vi "Test Read DAT and TDMS.vi"() -> ()   [LabVIEW 2019]
uses:
  3811ab8e-563b-4f0e-ab82-2145b4b5b4ca.vi
  9b17270d-5d0c-4365-9a1f-7ea8eb203ad9.vi
  6996a507-959e-4011-8723-71fb57f9d81e.vi
  06af5cf2-6c13-4970-920c-06c6a4bda324.vi
  0d41830b-9568-4bf9-b5e1-5d65a9571d75.vi
  1d0c72e7-2fd5-4ada-9d2c-d8c7b4a58351.vi
  <userlib>/_OpenG.lib/file/file.llb/Build Path - File Names Array__ogtk.vi
  <vilib>/Utility/error.llb/Error Cluster From Error Code.vi
  LV-Data/LV-Data.lvclass
panel:
  in  "TDMS Folder":path=path "G:/.shortcut-targets-by-id/0B8-gGFa6hkR4XzJJMDlqZXVKRk0/ansom/Data/MNK/SA40379A.20221206/01 - Vtg test"
  in  "TDMS File":path=path "G:/.shortcut-targets-by-id/0B8-gGFa6hkR4XzJJMDlqZXVKRk0/ansom/Data/PPMSDAQ/2020/PPMS 1/SA40244A.20210723/03-Sweep B IV/SA40244A.20210723.000000.tdms"
  in  "DAT file":path=path "G:/.shortcut-targets-by-id/0B8-gGFa6hkR4XzJJMDlqZXVKRk0/ansom/Data/MNK/SA40286K.20220307/00-Cooldown/SA40286K.20220307.000000.dat"
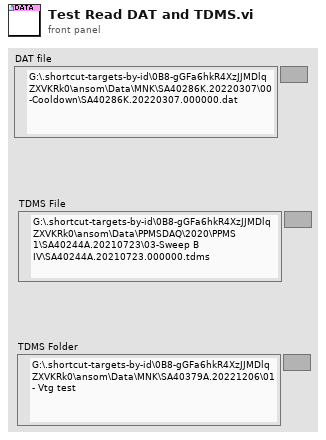
[diagram p1: front panel]
types:
  T1 = typedef "LV-Data.lvclass/Dictionary--cluster.ctl" = cluster{"key":string, "value":variant}
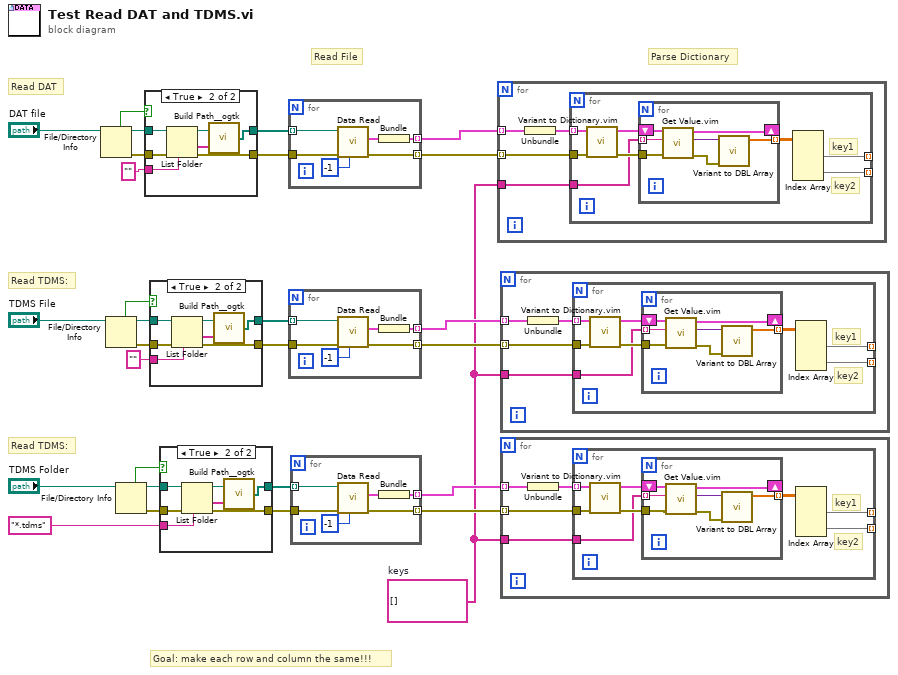
[diagram p0: block diagram]
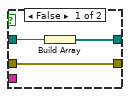
[diagram p2: hidden frame]
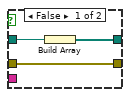
[diagram p3: hidden frame]
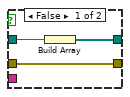
[diagram p4: hidden frame]
diagram:
  w16 = string[] []  # keys
  # "Goal: make each row and column the same!!!"
  # "Parse Dictionary"
  # "Read File"
  # "Read DAT"
  # "Read TDMS:"
  # "Read TDMS:"
  n1 = File/Directory Info(path="DAT file") -> (path out=w10:path, directory=w8:bool, error out=w9:errorcluster)  [unwired: 1 in, 4 out]
  n2 = File/Directory Info(path="TDMS File") -> (path out=w12:path, directory=w14:bool, error out=w13:errorcluster)  [unwired: 1 in, 4 out]
  n3 = File/Directory Info(path="TDMS Folder") -> (path out=w27:path, directory=w15:bool, error out=w25:errorcluster)  [unwired: 1 in, 4 out]
  n4 = case shown="True" w8 {
    tunnel: w10 -> [w31 w38]
    tunnel: [w30 w37] -> w5
    tunnel: w9 -> [w29 w36]
    tunnel: [w29 w35] -> w4
    tunnel: "" ("pattern") -> [_ w34]
    frame False {
      n5 = Build Array(w31) -> (w30:path[])
    }
    frame True {
      n6 = List Folder(path=w38, pattern=w34, error in=w36) -> (path out=w33:path, folder names=w32:string[], error out=w35:errorcluster)  [unwired: 1 in, 1 out]
      n7 = call-poly <userlib>:"Build Path__ogtk.vi"("name or relative path"=w32, "base path"=w33) -> ("appended path"=w37:path[])
    }
  }
  n8 = case shown="True" w14 {
    tunnel: w12 -> [w41 w48]
    tunnel: [w40 w47] -> w11
    tunnel: w13 -> [w39 w46]
    tunnel: [w39 w45] -> w3
    tunnel: "" ("pattern") -> [_ w44]
    frame False {
      n9 = Build Array(w41) -> (w40:path[])
    }
    frame True {
      n10 = List Folder(path=w48, pattern=w44, error in=w46) -> (path out=w43:path, folder names=w42:string[], error out=w45:errorcluster)  [unwired: 1 in, 1 out]
      n11 = call-poly <userlib>:"Build Path__ogtk.vi"("name or relative path"=w42, "base path"=w43) -> ("appended path"=w47:path[])
    }
  }
  n12 = case shown="True" w15 {
    tunnel: w27 -> [w51 w58]
    tunnel: [w50 w57] -> w26
    tunnel: w25 -> [w49 w56]
    tunnel: [w49 w55] -> w24
    tunnel: "*.tdms" ("pattern") -> [_ w54]
    frame False {
      n13 = Build Array(w51) -> (w50:path[])
    }
    frame True {
      n14 = List Folder(path=w58, pattern=w54, error in=w56) -> (path out=w53:path, folder names=w52:string[], error out=w55:errorcluster)  [unwired: 1 in, 1 out]
      n15 = call-poly <userlib>:"Build Path__ogtk.vi"("name or relative path"=w52, "base path"=w53) -> ("appended path"=w57:path[])
    }
  }
  n16 = for {
    tunnel: w5 -> [w64] mode=indexing
    tunnel: [w61] -> w17 mode=indexing
    tunnel: [w60] -> w18 mode=indexing
    tunnel: w4 -> [w59]
    n17 = call "Data Read.vi"("Append Index"=-1, "error in (no error)"=w59, "path"=w64) -> ("error out"=w60:errorcluster, "Data (Dictionary)"=w62:T1[])  [unwired: 5 in, 2 out]
    n18 = Bundle("Data (Dictionary)"=w62) -> (w61:cluster{"Data (Dictionary)":T1[]})  [unwired: 1 in]
  }
  n19 = for {
    tunnel: w11 -> [w70] mode=indexing
    tunnel: [w67] -> w19 mode=indexing
    tunnel: [w66] -> w20 mode=indexing
    tunnel: w3 -> [w65]
    n20 = call "Data Read.vi"("Append Index"=-1, "error in (no error)"=w65, "path"=w70) -> ("error out"=w66:errorcluster, "Data (Dictionary)"=w68:T1[])  [unwired: 5 in, 2 out]
    n21 = Bundle("Data (Dictionary)"=w68) -> (w67:cluster{"Data (Dictionary)":T1[]})  [unwired: 1 in]
  }
  n22 = for {
    tunnel: w26 -> [w76] mode=indexing
    tunnel: w24 -> [w75]
    tunnel: [w73] -> w22 mode=indexing
    tunnel: [w71] -> w21 mode=indexing
    n23 = call "Data Read.vi"("Append Index"=-1, "error in (no error)"=w75, "path"=w76) -> ("error out"=w71:errorcluster, "Data (Dictionary)"=w72:T1[])  [unwired: 5 in, 2 out]
    n24 = Bundle("Data (Dictionary)"=w72) -> (w73:cluster{"Data (Dictionary)":T1[]})  [unwired: 1 in]
  }
  n25 = for {
    tunnel: w17 -> [w80] mode=indexing
    tunnel: w18 -> [w78] mode=indexing
    tunnel: w16 -> [w77]
    n26 = Unbundle(w80) -> ("Data (Dictionary)"=w79:T1[])
    n27 = for {
      tunnel: w79 -> [w87] mode=indexing
      tunnel: [w85] -> _ mode=indexing
      tunnel: [w84] -> _ mode=indexing
      tunnel: w78 -> [w83]
      tunnel: w77 -> [w81]
      # "key2"
      # "key1"
      n28 = call "Variant to Dictionary.vim"("error in (no error)"=w83, "key-value"=w87) -> ("error out"=w82:errorcluster, "Dictionary"=w88:T1[])  [unwired: 8 in]
      n29 = for {
        tunnel: w81 -> [w93] mode=indexing
        shift-right: [w91] -> _
        shift-left: w88 -> [w92]
        tunnel: [w90] -> w86 mode=indexing
        tunnel: w82 -> [w89]
        n30 = call "Get Value.vim"("error in (no error)"=w89, "Key"=w93, "map in"=w92) -> ("error out"=w94:errorcluster, "value"=w95:variant, "map out"=w91:T1[])  [unwired: 6 in]
        n31 = call "Variant to DBL Array.vi"("error in (no error)"=w94, "Data (Variant)"=w95) -> ("1D Array"=w90:dbl[])  [unwired: 7 in, 2 out]
      }
      n32 = Index Array(array=w86) -> (element #1=w85:dbl[], element #2=w84:dbl[])  [unwired: 4 in]
    }
  }
  n33 = for {
    tunnel: w19 -> [w99] mode=indexing
    tunnel: w20 -> [w97] mode=indexing
    tunnel: w16 -> [w96]
    n34 = Unbundle(w99) -> ("Data (Dictionary)"=w98:T1[])
    n35 = for {
      tunnel: w98 -> [w106] mode=indexing
      tunnel: [w104] -> _ mode=indexing
      tunnel: [w103] -> _ mode=indexing
      tunnel: w97 -> [w102]
      tunnel: w96 -> [w100]
      # "key2"
      # "key1"
      n36 = call "Variant to Dictionary.vim"("error in (no error)"=w102, "key-value"=w106) -> ("error out"=w101:errorcluster, "Dictionary"=w107:T1[])  [unwired: 8 in]
      n37 = for {
        tunnel: w100 -> [w112] mode=indexing
        shift-right: [w110] -> _
        shift-left: w107 -> [w111]
        tunnel: [w109] -> w105 mode=indexing
        tunnel: w101 -> [w108]
        n38 = call "Get Value.vim"("error in (no error)"=w108, "Key"=w112, "map in"=w111) -> ("error out"=w113:errorcluster, "value"=w114:variant, "map out"=w110:T1[])  [unwired: 6 in]
        n39 = call "Variant to DBL Array.vi"("error in (no error)"=w113, "Data (Variant)"=w114) -> ("1D Array"=w109:dbl[])  [unwired: 7 in, 2 out]
      }
      n40 = Index Array(array=w105) -> (element #1=w104:dbl[], element #2=w103:dbl[])  [unwired: 4 in]
    }
  }
  n41 = for {
    tunnel: w16 -> [w115]
    tunnel: w22 -> [w118] mode=indexing
    tunnel: w21 -> [w116] mode=indexing
    n42 = Unbundle(w118) -> ("Data (Dictionary)"=w117:T1[])
    n43 = for {
      tunnel: w115 -> [w119]
      tunnel: w117 -> [w125] mode=indexing
      tunnel: [w123] -> _ mode=indexing
      tunnel: [w122] -> _ mode=indexing
      tunnel: w116 -> [w121]
      # "key2"
      # "key1"
      n44 = call "Variant to Dictionary.vim"("error in (no error)"=w121, "key-value"=w125) -> ("error out"=w120:errorcluster, "Dictionary"=w126:T1[])  [unwired: 8 in]
      n45 = for {
        tunnel: w119 -> [w131] mode=indexing
        shift-right: [w129] -> _
        shift-left: w126 -> [w130]
        tunnel: [w128] -> w124 mode=indexing
        tunnel: w120 -> [w127]
        n46 = call "Get Value.vim"("error in (no error)"=w127, "Key"=w131, "map in"=w130) -> ("error out"=w132:errorcluster, "value"=w133:variant, "map out"=w129:T1[])  [unwired: 6 in]
        n47 = call "Variant to DBL Array.vi"("error in (no error)"=w132, "Data (Variant)"=w133) -> ("1D Array"=w128:dbl[])  [unwired: 7 in, 2 out]
      }
      n48 = Index Array(array=w124) -> (element #1=w123:dbl[], element #2=w122:dbl[])  [unwired: 4 in]
    }
  }
